vi "Measurement Logic.vi"() -> ()   [LabVIEW 2024, in "Dynamic Signal Acquisition (Interactive).lvlib"]
uses:
  Dynamic Signal Acquisition (Interactive).lvlib
  <vilib>/Plug-In SDKs/Measurements/Measure Call Context/Measure Call Context.lvclass
  Measurement Configuration.ctl
  <vilib>/Addons/_XControls/Numeric with String Overlay/Numeric with String Overlay.xctl
  <extravilib>/ChannelInstances/Tag-bool/Instantiate.vi
  <extravilib>/ChannelInstances/Event Messenger-bool/Instantiate.vi
  Dynamic Signal Acquisition (Interactive) UI/Dynamic Signal Acquisition (Interactive) UI.lvlib
  Measurement Results.ctl
panel:
  out "measurement results":T1
  in  "measurement configuration":T2={"DAQmx configuration json"="", "window"=1, "overlap"=32.0, "averaging mode"=64, "number of averages"=64.0} {"averaging mode" items=["No averaging", "Vector averaging", "RMS averaging", "Peak hold"]; "window" items=["None "=0, "Hanning"=1, "Flat Top"=6, "7 Term B-Harris"=8]}
  out "measure call context out":refnum<class "Measure Call Context.lvclass">
  in  "measure call context in":refnum<class "Measure Call Context.lvclass">
  out "error out":errorcluster
  in  "error in":errorcluster
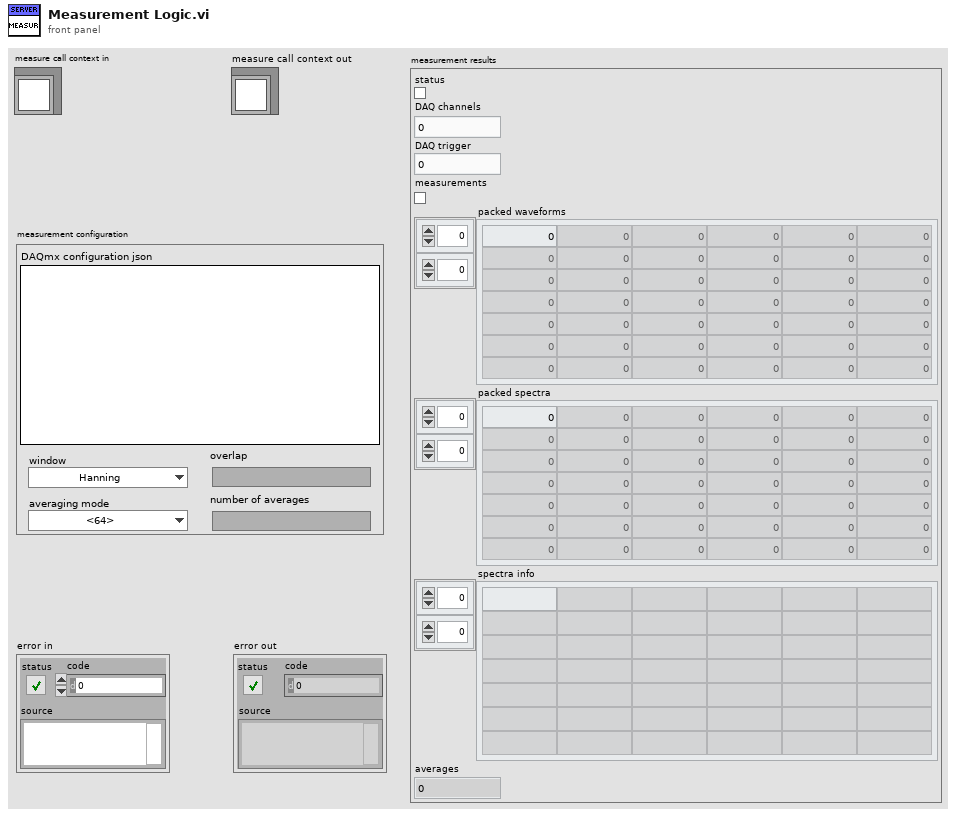
[diagram p1: front panel]
types:
  T1 = typedef "Dynamic Signal Acquisition (Interactive).lvlib/Measurement Results.ctl" = cluster{"status":bool, "DAQ channels":u32, "DAQ trigger":u32, "measurements":bool, "packed waveforms":dbl[][], "packed spectra":dbl[][], "spectra info":string[][], "averages":dbl}
  T2 = typedef "Dynamic Signal Acquisition (Interactive).lvlib/Measurement Configuration.ctl" = cluster{"DAQmx configuration json":string, "window":u32, "overlap":dbl, "averaging mode":u32, "number of averages":dbl}
  T3 = enum16{"No averaging", "Vector averaging", "RMS averaging", "Peak hold"}
  T4 = cluster{"averaging mode":enum16{"No averaging", "Vector averaging", "RMS averaging", "Peak hold"}, "weighting mode":enum16{"Linear", "Exponential"}, "number of averages":u32, "linear mode":enum16{"One shot", "Auto restart"}}
  T5 = typedef "Dynamic Signal Acquisition (Interactive) UI.lvlib/SFPDAQ Configuration.ctl" = cluster{"Run Mode":u16, "Sample Rate (Hz)":dbl, "Block Size":i32, "Channel Table":T6[], "Trigger Type":u16, "Trigger Channel":string, "Level":dbl, "Pretrigger":i32, "Hysteresis":dbl, "Slope":enum16{"Falling", "Rising"}}
  T6 = typedef "Dynamic Signal Acquisition (Interactive) UI.lvlib/SFPDAQmx Channel Info.ctl" = cluster{"DAQmx Channel":tag, "Channel Type":u16, "Max":dbl, "Sensitivity":dbl, "Coupling":enum16{"AC", "DC"}, "input terminal configuration":i32, "excitation":enum16{"Off", "Min", "Max"}}
  T7 = typedef "Tag-bool.lvlib/))Channel.ctl" = refnum<queue>
  T8 = typedef "Event Messenger-bool.lvlib/))Channel.ctl" = refnum<queue>
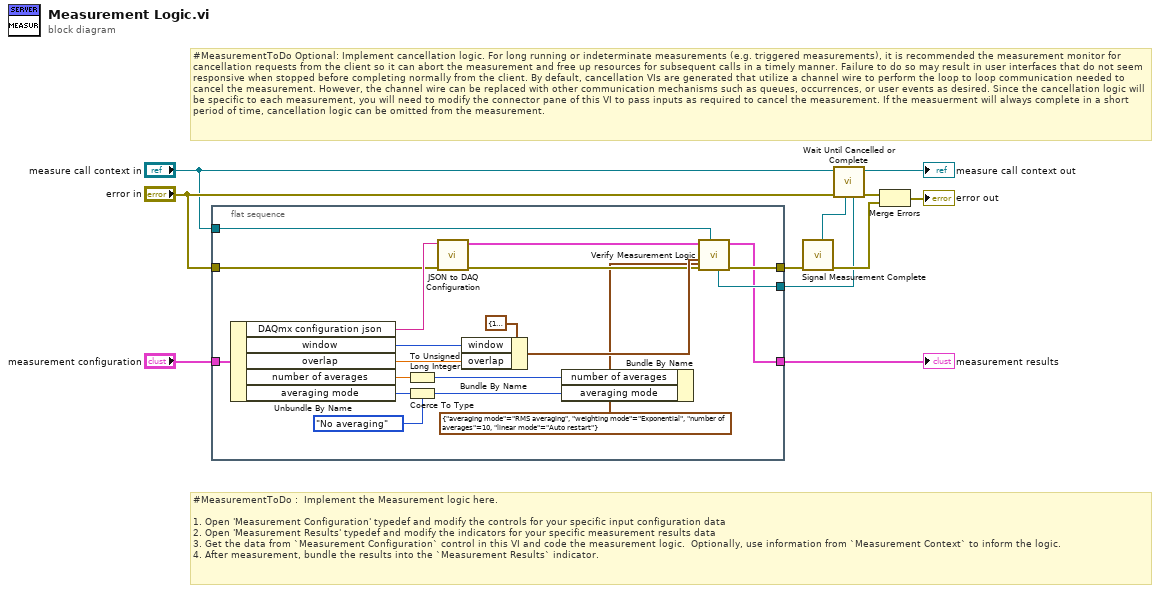
[diagram p0: block diagram]
diagram:
  # "#MeasurementToDo Optional: Implement cancellation logic. For long running or indeterminate measurements (e.g. triggered measurements), it is recommended the measurement monitor for cancellation requests from the client so it can abort the measurement and free up resources for subsequent calls in a timely manner. Failure to do so may result in user interfaces that do not seem responsive when stopped before completing normally from the client. By default, cancellation VIs are generated that utilize a channel wire to perform the loop to loop communication needed to cancel the measurement. However, the channel wire can be replaced with other communication mechanisms such as queues, occurrences, or user events as desired. Since the cancellation logic will be specific to each measurement, you will need to modify the connector pane of this VI to pass inputs as required to cancel the measurement. If the measuerment will always complete in a short period of time, cancellation logic can be omitted from the measurement."
  # "#MeasurementToDo :  Implement the Measurement logic here.\n\n1. Open 'Measurement Configuration' typedef and modify the controls for your specific input configuration data\n2. Open 'Measurement Results' typedef and modify the indicators for your specific measurement results data\n3. Get the data from `Measurement Configuration` control in this VI and code the measurement logic.  Optionally, use information from `Measurement Context` to inform the logic.\n4. After measurement, bundle the results into the `Measurement Results` indicator."
  n1 = flat-sequence {
    tunnel: "measurement configuration" -> [w30]
    tunnel: [w12] -> w10
    tunnel: "error in" -> [w18]
    tunnel: [w21] -> w7
    tunnel: "measure call context in" -> [w16]
    tunnel: [w14] -> w1
    frame #0 {
      w13 = T4 {"averaging mode"=enum."RMS averaging", "weighting mode"=enum."Exponential", "number of averages"=10, "linear mode"=enum."Auto restart"} ("averaging parameters")
      n2 = Unbundle By Name(w30) -> ("DAQmx configuration json"=w19:string, "window"=w22:u32, "overlap"=w28:dbl, "number of averages"=w27:dbl, "averaging mode"=w25:u32)
      n3 = To Unsigned Long Integer(number=w27) -> (unsigned 32bit integer=w26:u32)
      n4 = Coerce To Type(0:w25, 1:T3."No averaging" ("averaging mode")) -> (2:w23:T3)
      n5 = call "JSON to DAQ Configuration.vi"("error in"=w18, "flattened JSON configuration"=w19) -> ("error out"=w17:errorcluster, "DAQmx Configuration"=w15:T5)  [unwired: 8 in]
      n6 = Bundle By Name(cluster=cluster{"window":u32, "overlap":dbl} {"window"=1, "overlap"=32.0} ("window and overlap"), "window"=w22, "overlap"=w28) -> (w20:cluster{"window":u32, "overlap":dbl})
      n7 = Bundle By Name(cluster=w13, "number of averages"=w26, "averaging mode"=w23) -> ()  [unwired: 1 out]
      n8 = call "Verify Measurement Logic.vi"("averaging parameters"=w13, "Measure Call Context in"=w16, "error in"=w17, "window and overlap"=w20, "DAQmx Configuration"=w15) -> ("error out"=w21:errorcluster, "last measurement results"=w12:T1, "stop channel"=w14:T7)  [unwired: 4 in]
    }
  }
  n9 = call "Signal Measurement Complete.vi"("error in (no error)"=w7) -> ("error out"=w5:errorcluster, "done channel"=w6:T8)  [unwired: 9 in]
  n10 = call "Wait Until Cancelled or Complete.vi"("stop channel"=w1, "done channel"=w6, "error in (no error)"="error in", "measure call context in"="measure call context in") -> ("error out"=w4:errorcluster, "measure call context out"=→"measure call context out":refnum<class "Measure Call Context.lvclass">)  [unwired: 6 in]
  n11 = Merge Errors(w4, w5) -> (→"error out":errorcluster)
  "measurement results" <- w10
